vi "Initialize.vi"(5 "RS485-Address (128: RS232)":u8=128, 7 "Serial Configuration":T1={"Baud Rate"=4800, "Parity"=2, "Data Bits"=7, "Stop Bits"=10, "Flow Control"=2} {"Flow Control" items=["None", "XON/XOFF", "RTS/CTS", "XON/XOFF & RTS/CTS", "DTR/DSR", "XON/XOFF & DTR/DSR"]; "Stop Bits" items=["1.0"=10, "1.5"=15, "2.0"=20]; "Data Bits" items=["7"=7, "8"=8]; "Parity" items=["None", "Odd", "Even", "Mark", "Space"]; "Baud Rate" items=["300"=300, "600"=600, "1200"=1200, "2400"=2400, "4800"=4800, "9600"=9600, "19200"=19200]}, 8 "error in (no error)":errorcluster, 9 "Reset / Default (T: Both)":bool=TRUE, 10 "ID Query? (T: Yes)":bool=TRUE, 11 "VISA resource name":refnum<visa-resource-name>) -> (0 "error out":errorcluster, 3 "VISA resource name out":refnum<visa-resource-name>)   [LabVIEW 2018, in "JULABO DeviceDriver.lvlib"]
doc: "Establishes communication with the instrument and optionally performs an instrument identification query and/or an instrument reset. It also places the instrument in a default state needed for other instrument driver operations. Therefore, call this VI before calling other instrument driver VIs for this instrument. Generally, you need to call the <B>Initialize VI</B> only once at the beginning of an application."
uses:
  JULABO DeviceDriver.lvlib
panel:
  out "AnswerString (output)":string
  # "© 2010 <JULABO Labortechnik GmbH>.  ALL RIGHTS RESERVED."
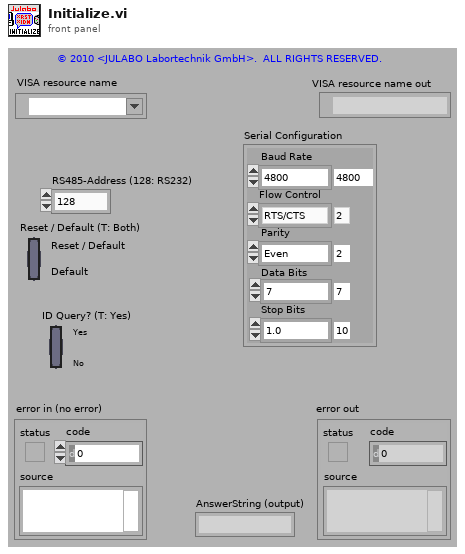
[diagram p1: front panel]
types:
  T1 = cluster{"Baud Rate":u32, "Parity":u16, "Data Bits":u16, "Stop Bits":u16, "Flow Control":u16}
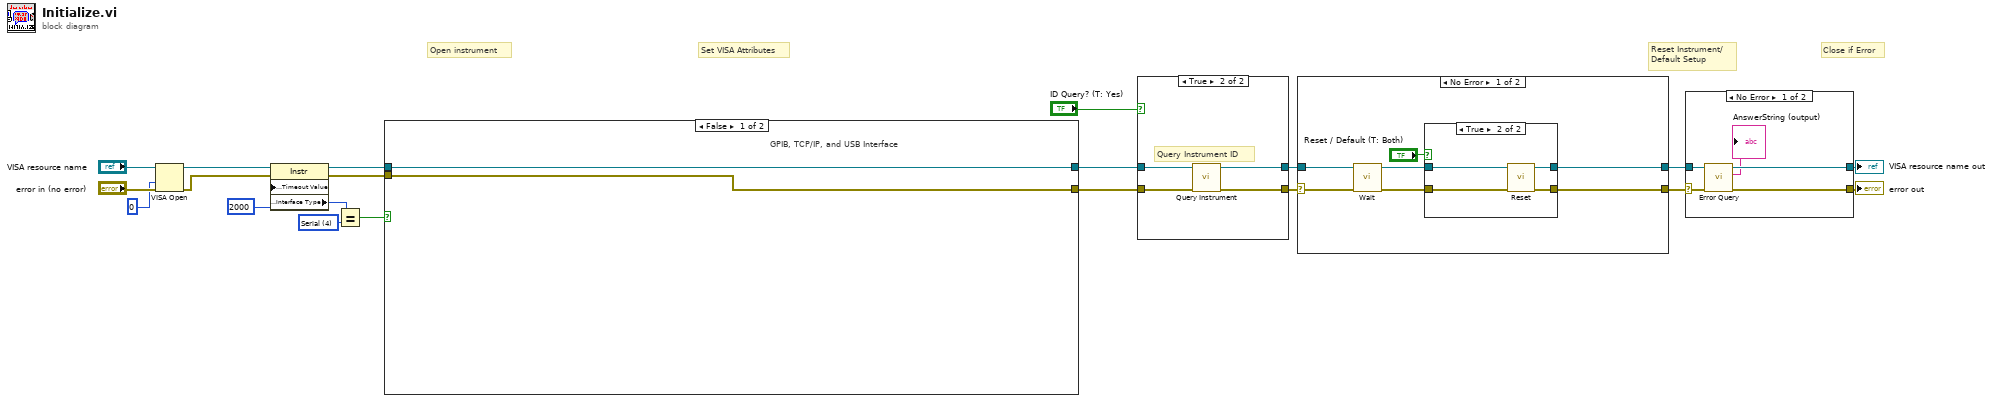
[diagram p0: block diagram]
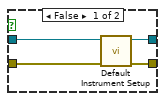
[diagram p3: hidden frame]
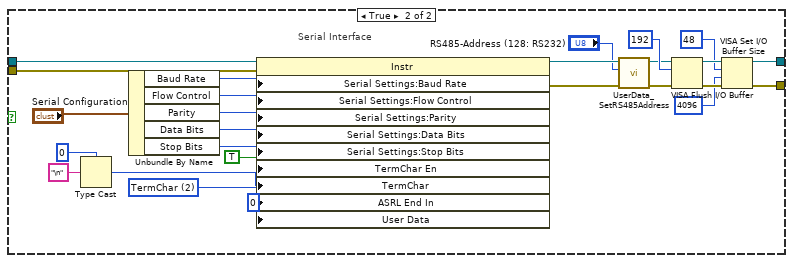
[diagram p5: hidden frame]
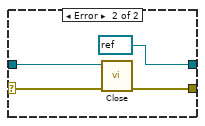
[diagram p6: hidden frame]
diagram:
  w11 = u16 4 items=["GPIB"=1, "VXI"=2, "GPIB-VXI"=3, "Serial"=4, "PXI"=5, "TCPIP"=6, "USB"=7] ("Interface Information:Interface Type")
  # "Set VISA Attributes"
  # "Close if Error"
  # "Reset Instrument/\nDefault Setup"
  # "Open instrument"
  n1 = VISA Open(access mode=u32 0, error in (no error)="error in (no error)", VISA resource name="VISA resource name") -> (VISA resource name=w2:refnum<visa-resource-name>, error out=w1:errorcluster)  [unwired: 2 in]
  n2 = property class="Instr"(reference=w2, error in=w1, "General Settings:Timeout Value"=u32 2000) -> (reference out=w14:refnum<visa-resource-name>, error out=w13:errorcluster, "Interface Information:Interface Type"=w18:u16)
  n3 = Equal?(x=w18, y=w11) -> (x = y?=w12:bool)
  n4 = case shown="False" w12 {
    tunnel: [w21 w46] -> w16
    tunnel: [w22 w45] -> w15
    tunnel: w14 -> [w21 w47]
    tunnel: w13 -> [w22 w48]
    frame False {
      # "GPIB, TCP/IP, and USB Interface"
    }
    frame True {
      w34 = u16 2 items=["None", "Last Bit", "TermChar"] ("Serial Settings:End Mode for Reads")
      # "Serial Interface"
      n5 = Type Cast(type=u8 0, x="\n") -> (*(type *) &x=w35:u8)
      n6 = Unbundle By Name("Serial Configuration") -> ("Baud Rate"=w43:u32, "Flow Control"=w39:u16, "Parity"=w41:u16, "Data Bits"=w42:u16, "Stop Bits"=w38:u16)
      n7 = property class="Instr"(reference=w47, error in=w48, "Serial Settings:Baud Rate"=w43, "Serial Settings:Flow Control"=w39, "Serial Settings:Parity"=w41, "Serial Settings:Data Bits"=w42, "Serial Settings:Stop Bits"=w38, "TermChar En"=TRUE ("Message Based Settings:Termination Character Enable"), "TermChar"=w35, "ASRL End In"=w34, "User Data"=u32 0 ("General Settings:User Data")) -> (reference out=w26:refnum<visa-resource-name>, error out=w25:errorcluster)
      n8 = call "UserData_SetRS485Address.vi"("Fehler (Eingang)"=w25, "Address (128:RS232)"="RS485-Address (128: RS232)", "VISA resource name in"=w26) -> ("Fehler (Ausgang)"=w27:errorcluster, "VISA resource name out"=w28:refnum<visa-resource-name>)  [unwired: 3 in]
      n9 = VISA Flush I/O Buffer(VISA resource name=w28, mask (16)=u16 192, error in (no error)=w27) -> (VISA resource name out=w33:refnum<visa-resource-name>, error out=w32:errorcluster)
      n10 = VISA Set I/O Buffer Size(VISA resource name=w33, mask (16)=u16 48, size (4096)=u32 4096 ("size (0)"), error in (no error)=w32) -> (VISA resource name out=w46:refnum<visa-resource-name>, error out=w45:errorcluster)
    }
  }
  n11 = case shown="True" "ID Query? (T: Yes)" {
    tunnel: w16 -> [w50 w54]
    tunnel: w15 -> [w49 w53]
    tunnel: [w49 w52] -> w7
    tunnel: [w50 w51] -> w6
    frame False {
    }
    frame True {
      # "Query Instrument ID"
      n12 = call "Query Instrument.vi"("error in"=w53, "VISA resource name (Eingang)"=w54) -> ("error out"=w52:errorcluster, "VISA resource name (Ausgang)"=w51:refnum<visa-resource-name>)  [unwired: 6 in, 2 out]
    }
  }
  n13 = case shown="No Error" w7 {
    selector: w7 -> [w56 w70]
    tunnel: [w60 w70] -> w4
    tunnel: [w59 w71] -> w5
    tunnel: w6 -> [w61 w71]
    frame No Error {
      n14 = call "Wait.vi"("error in"=w56, "VISA resource name in"=w61) -> ("error out"=w55:errorcluster, "VISA resource name out"=w57:refnum<visa-resource-name>)  [unwired: 4 in]
      n15 = case shown="True" "Reset / Default (T: Both)" {
        tunnel: w55 -> [w62 w66]
        tunnel: [w63 w69] -> w60
        tunnel: w57 -> [w65 w67]
        tunnel: [w64 w68] -> w59
        frame False {
          n16 = call "Default Instrument Setup.vi"("error in (no error)"=w62, "VISA resource name"=w65) -> ("error out"=w63:errorcluster, "VISA resource name out"=w64:refnum<visa-resource-name>)  [unwired: 8 in]
        }
        frame True {
          n17 = call "Reset.vi"("error in (no error)"=w66, "VISA resource name"=w67) -> ("error out"=w69:errorcluster, "VISA resource name out"=w68:refnum<visa-resource-name>)  [unwired: 8 in]
        }
      }
    }
    frame Error {
    }
  }
  n18 = case shown="No Error" w4 {
    selector: w4 -> [w74 w78]
    tunnel: w5 -> [w73 w79]
    tunnel: [w76 refnum<visa-resource-name> refnum ("VISA resource name out")] -> w9
    tunnel: [w75 w80] -> w8
    frame No Error {
      n19 = call "Error Query.vi"("error in (no error)"=w74, "VISA resource name"=w73) -> ("error out"=w75:errorcluster, "AnswerString (output)"=→"AnswerString (output)":string, "VISA resource name out"=w76:refnum<visa-resource-name>)  [unwired: 6 in, 1 out]
    }
    frame Error {
      n20 = call "Close.vi"("error in (no error)"=w78, "VISA resource name"=w79) -> ("error out"=w80:errorcluster)  [unwired: 9 in]
    }
  }
  "VISA resource name out" <- w9
  "error out" <- w8
